vi "Panel.vi"(11 "AudioMonPanel in":refnum<class "AudioMonPanel.lvclass">) -> ()   [LabVIEW 2022 SP3, in "TouchControl.lvlib" / "AudioMonPanel.lvclass"]
uses:
  AudioMonPanel.lvclass
  C:/Program Files (x86)/National Instruments/LabVIEW 2022/vi.lib/IlluminatedG/IG OOPanel/OOPanel/Panel/Panel.lvclass
  <vilib>/IlluminatedG/IG OOPanel/OOPanel/Panel/Basic UI State.ctl
  VMR Server Shared/Audio Summary.ctl
  VMR Server Shared/Channel.ctl
  <vilib>/IlluminatedG/IG OOPanel/OOPanel/Panel/Panel.lvclass
  <vilib>/IlluminatedG/IG OOPanel/OOPanel/OOPanel.lvlib
  TouchControl.lvlib
  <vilib>/httpClient/LabVIEWHTTPClient.lvlib
  VMR Server Shared/VMR Server Shared.lvlib
panel:
  out "Meter 32":dbl(knob) scale=0.0..1.0
  out "Meter 31":dbl(knob) scale=0.0..1.0
  out "Meter 30":dbl(knob) scale=0.0..1.0
  out "Meter 29":dbl(knob) scale=0.0..1.0
  out "Meter 28":dbl(knob) scale=0.0..1.0
  out "Meter 27":dbl(knob) scale=0.0..1.0
  out "Meter 26":dbl(knob) scale=0.0..1.0
  out "Meter 25":dbl(knob) scale=0.0..1.0
  out "Meter 24":dbl(knob) scale=0.0..1.0
  out "Meter 23":dbl(knob) scale=0.0..1.0
  out "Meter 22":dbl(knob) scale=0.0..1.0
  out "Meter 21":dbl(knob) scale=0.0..1.0
  out "Meter 20":dbl(knob) scale=0.0..1.0
  out "Meter 19":dbl(knob) scale=0.0..1.0
  out "Meter 18":dbl(knob) scale=0.0..1.0
  out "Meter 17":dbl(knob) scale=0.0..1.0
  out "Meter 16":dbl(knob) scale=0.0..1.0
  out "Meter 15":dbl(knob) scale=0.0..1.0
  out "Meter 14":dbl(knob) scale=0.0..1.0
  out "Meter 13":dbl(knob) scale=0.0..1.0
  out "Meter 12":dbl(knob) scale=0.0..1.0
  out "Meter 11":dbl(knob) scale=0.0..1.0
  out "Meter 10":dbl(knob) scale=0.0..1.0
  out "Meter 9":dbl(knob) scale=0.0..1.0
  out "Meter 8":dbl(knob) scale=0.0..1.0
  out "Meter 7":dbl(knob) scale=0.0..1.0
  out "Meter 6":dbl(knob) scale=0.0..1.0
  out "Meter 5":dbl(knob) scale=0.0..1.0
  out "Meter 4":dbl(knob) scale=0.0..1.0
  out "Meter 3":dbl(knob) scale=0.0..1.0
  out "Meter 2":dbl(knob) scale=0.0..1.0
  out "Meter 1":dbl(knob) scale=0.0..1.0
  # "MIC IN"
  # "B"
  # "C"
  # "VBAN"
  # "MUSIC"
  # "DESKTOP"
  # "CHAT IN"
  # "AUX"
  # "SPEAKERS"
  # "PHONES"
  # "TV"
  # "MIC OUT"
  # "MUSIC"
  # "STREAM"
  # "CHAT OUT"
  # "VBAN OUT"
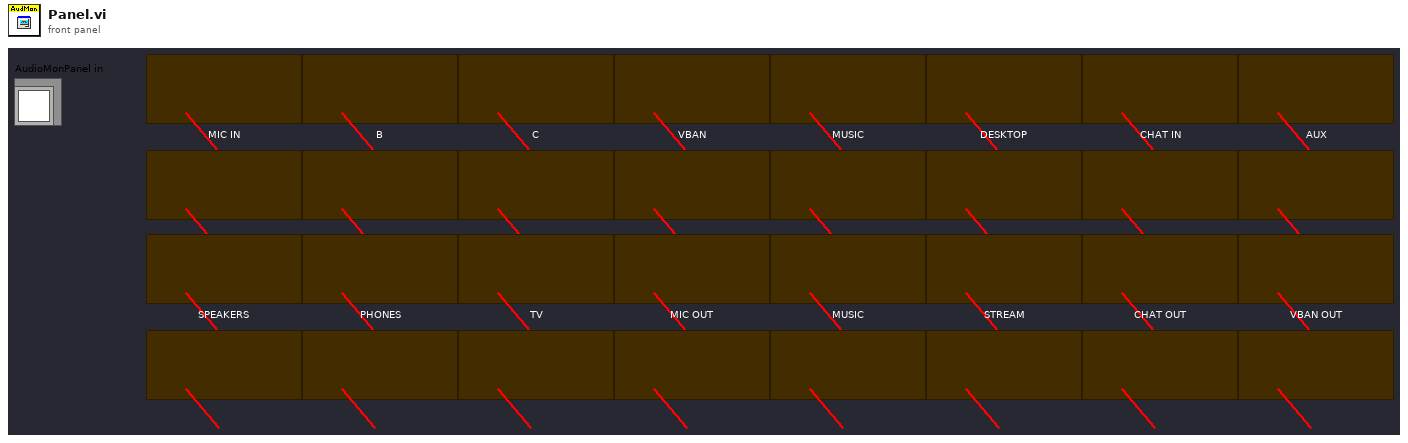
[diagram p1: front panel]
types:
  T1 = typedef "OOPanel.lvlib/Panel.lvclass/Basic UI State.ctl" = enum16{"Init", "Run", "Close"}
  T2 = typedef "VMR Server Shared.lvlib/Audio Summary.ctl" = cluster{"Route":bool[][], "Channels":T3[]}
  T3 = typedef "VMR Server Shared.lvlib/Channel.ctl" = cluster{"Gain":dbl, "Muted":bool, "Levels":cluster{"L":dbl, "R":dbl}}
  T4 = typedef "OOPanel.lvlib/Panel.lvclass/Panel Events.ctl" = cluster{"Visbility":refnum<user-event>, "Close":refnum<user-event>}
  T5 = typedef "OOPanel.lvlib/Visibility State.ctl" = enum16{"Idle", "Closed", "Hidden", "Visible", "Subpanel", "Hidden Subpanel"}
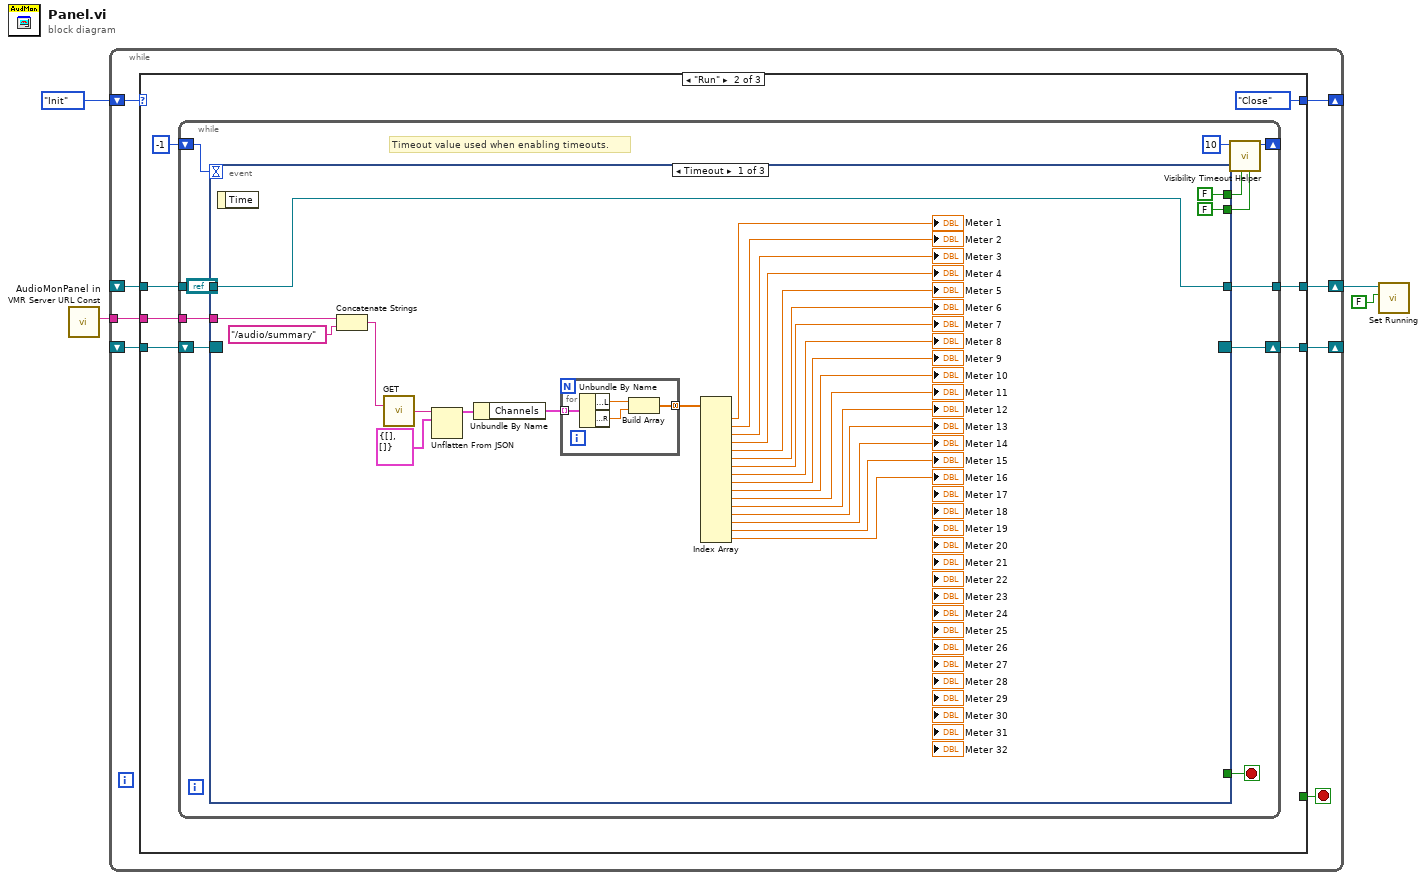
[diagram p0: block diagram]
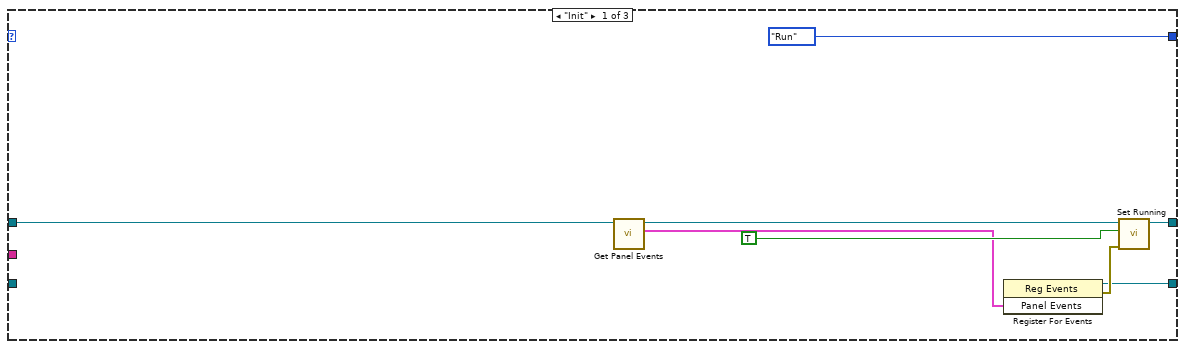
[diagram p2: hidden frame]
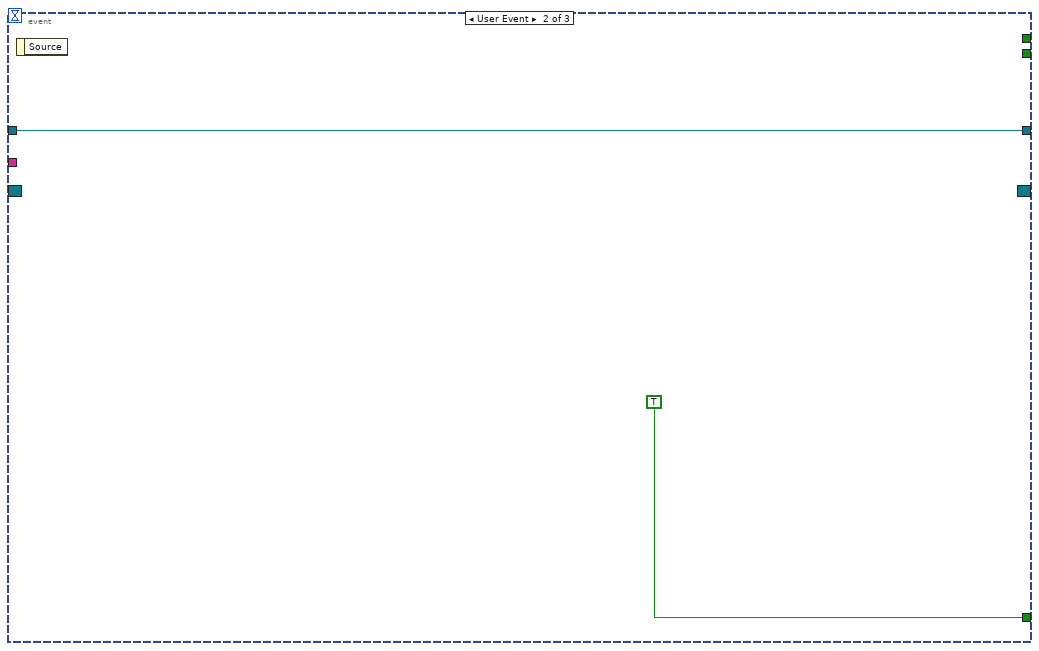
[diagram p3: hidden frame]
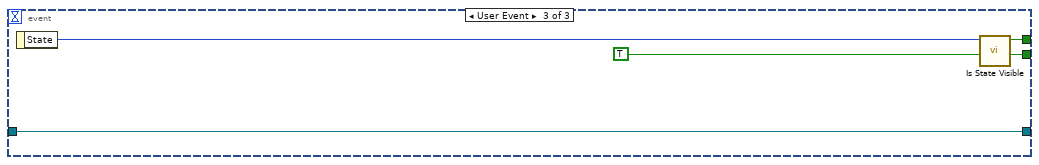
[diagram p4: hidden frame]
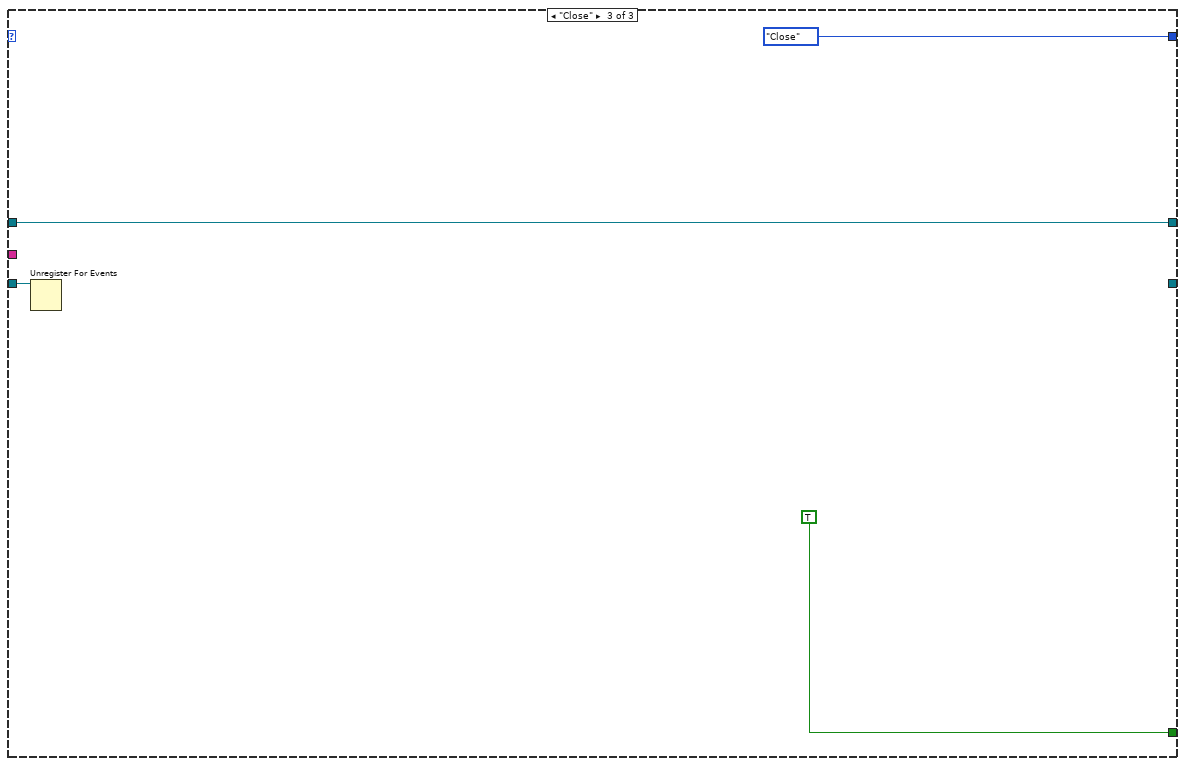
[diagram p5: hidden frame]
diagram:
  n1 = call "VMR Server URL Const.vi"() -> ("VMR Server URL"=w1:string)  [unwired: 11 in]
  n2 = while {
    shift-right: [w12] -> _
    shift-left: _ -> [w13]
    shift-right: [w10] -> _
    shift-left: Basic_UI_State."Init" ("Basic UI State") -> [w11]
    shift-right: [w8] -> w5
    shift-left: "AudioMonPanel in" -> [w7]
    tunnel: w1 -> [w6]
    stop <- w9 stop-if-true
    n3 = case shown="\"Run\"" w11 {
      tunnel: w13 -> [_ w28 w78]
      tunnel: [w18 w26 _] -> w12
      tunnel: [Basic_UI_State."Run" ("Basic UI State") Basic_UI_State."Close" ("Basic UI State") Basic_UI_State."Close" ("Basic UI State")] -> w10
      tunnel: [_ _ TRUE] -> w9
      tunnel: [w17 w23 w77] -> w8
      tunnel: w7 -> [w16 w24 w77]
      tunnel: w6 -> [_ w22 _]
      frame "Init" {
        n4 = call <vilib>:"Get Panel Events.vi"("Panel in"=w16) -> ("Panel Events"=w14:T4, "Panel out"=w15:refnum<class "AudioMonPanel.lvclass">)  [unwired: 8 in, 1 out]
        n5 = register-events(w14) -> (reference out=w18:refnum<event-registration>, error out=w20:errorcluster)  [unwired: 2 in]
        n6 = call <vilib>:"Set Running.vi"("error in (no error)"=w20, "Running"=TRUE, "Panel in"=w15) -> ("Panel out"=w17:refnum<class "AudioMonPanel.lvclass">)  [unwired: 7 in, 1 out]
      }
      frame "Run" {
        n7 = while {
          shift-right: [w35] -> w26
          shift-left: w28 -> [w36]
          shift-right: [w38] -> _
          shift-left: -1 ("Timeout") -> [w37]
          tunnel: w24 -> [w31]
          tunnel: [w30] -> w23
          tunnel: w22 -> [w29]
          stop <- w32 stop-if-true
          # "Timeout value used when enabling timeouts."
          n8 = event shown="[0] Timeout" {
            selector: w36 -> [_ _ _]
            dyn-events: [_ _ _] -> w35
            timeout: w37 -> [_ _ _]
            tunnel: [FALSE _ w75] -> w34
            tunnel: [FALSE _ TRUE] -> w33
            tunnel: [_ TRUE _] -> w32
            tunnel: w31 -> [w55 w71 w73]
            tunnel: [w55 w71 w73] -> w30
            tunnel: w29 -> [w64 _ _]
            event Timeout {
              n9 = event-data() -> ()  [unwired: 1 in, 1 out]
              n10 = Concatenate Strings(w64, "/audio/summary" ("string")) -> (w62:string)
              n11 = call <vilib>:"GET.vi"("url"=w62) -> ("body"=w61:string)  [unwired: 11 in, 3 out]
              n12 = Unflatten From JSON(JSON string=w61, type and defaults=T2 {"Route"=[], "Channels"=[]} ("Audio Summary")) -> (value=w59:T2)  [unwired: 5 in, 1 out]
              n13 = Unbundle By Name(w59) -> ("Channels"=w58:T3[])
              n14 = for {
                tunnel: w58 -> [w70] mode=indexing
                tunnel: [w67] -> w57 mode=concatenating
                n15 = Unbundle By Name(w70) -> ("Levels.L"=w69:dbl, "Levels.R"=w68:dbl)
                n16 = Build Array(w69, w68) -> (w67:dbl[])
              }
              n17 = Index Array(array=w57) -> (element #1=→"Meter 1":dbl, element #2=→"Meter 2":dbl, element #3=→"Meter 3":dbl, element #4=→"Meter 4":dbl, element #5=→"Meter 5":dbl, element #6=→"Meter 6":dbl, element #7=→"Meter 7":dbl, element #8=→"Meter 8":dbl, element #9=→"Meter 9":dbl, element #10=→"Meter 10":dbl, element #11=→"Meter 11":dbl, element #12=→"Meter 12":dbl, element #13=→"Meter 13":dbl, element #14=→"Meter 14":dbl, element #15=→"Meter 15":dbl, element #16=→"Meter 16":dbl)  [unwired: 16 in]
            }
            event User Event {
              n18 = event-data() -> ()  [unwired: 1 in, 1 out]
            }
            event User Event {
              n19 = event-data() -> ("State"=w76:T5)  [unwired: 1 in]
              n20 = call <vilib>:"Is State Visible.vi"("Visibility"=w76) -> ("Visible"=w75:bool)  [unwired: 10 in]
            }
          }
          n21 = call <vilib>:"Visibility Timeout Helper.vi"("Update?"=w33, "Use Timeout?"=w34, "Visible Timeout mS"=10) -> ("Timeout"=w38:i32)  [unwired: 8 in]
        }
      }
      frame "Close" {
        n22 = Unregister For Events(event registration refnum=w78) -> ()  [unwired: 1 in, 1 out]
      }
    }
  }
  n23 = call <vilib>:"Set Running.vi"("Running"=FALSE, "Panel in"=w5) -> ()  [unwired: 8 in, 2 out]
